vi "例4-29（2）.vi"() -> ()   [LabVIEW 2019]
panel:
  in  "停止":bool
  out "波形图表":T1(graph)
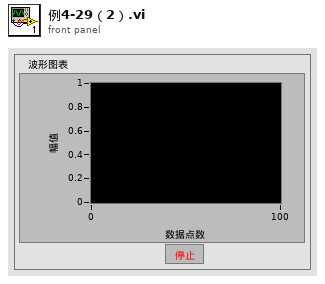
[diagram p1: front panel]
types:
  T1 = cluster{"number: 0 to 1":dbl, "number: 0 to 1":dbl}[]
  T2 = cluster{"number: 0 to 1":dbl, "number: 0 to 1":dbl}
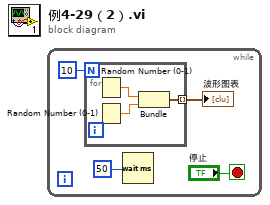
[diagram p0: block diagram]
diagram:
  n1 = while {
    stop <- "停止" stop-if-true
    n2 = for {
      N: 10 -> [_]
      tunnel: [w5] -> w1 mode=indexing
      n3 = Random Number (0-1)() -> (number: 0 to 1=w6:dbl)
      n4 = Random Number (0-1)() -> (number: 0 to 1=w7:dbl)
      n5 = Bundle("number: 0 to 1"=w6, "number: 0 to 1"=w7) -> (w5:T2)  [unwired: 1 in]
    }
    "波形图表" <- w1
    n6 = Wait (ms)(milliseconds to wait=50) -> ()  [unwired: 1 out]
  }
